vi "mqttCmdSend.vi"(0 "mqttBrokerCommand in":refnum<class "mqttCmd.lvclass">, 5 "byte1":u8, 7 "mqtt in":refnum<class "mqtt.lvclass">, 11 "error in (no error)":errorcluster) -> (4 "mqttBrokerCommand out":refnum<class "mqttCmd.lvclass">, 15 "error out":errorcluster)   [LabVIEW 2014, in "labview-mqtt.lvlib" / "mqttCmd.lvclass"]
uses:
  mqttCmd.lvclass
  mqtt.lvclass
  labview-mqtt.lvlib
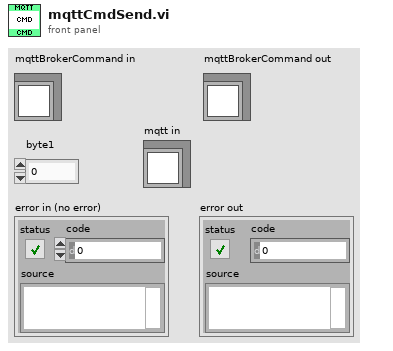
[diagram p1: front panel]
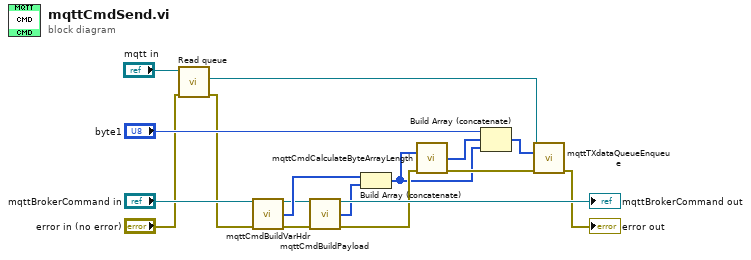
[diagram p0: block diagram]
diagram:
  n1 = call-dynamic "Read queue.vi"("error in (no error)"="error in (no error)", "mqtt in"="mqtt in") -> ("error out"=w1:errorcluster, "queue"=w3:refnum<queue>)  [unwired: 7 in, 1 out]
  n2 = call-dynamic "mqttCmdBuildVarHdr.vi"("_mqtt in"="mqttBrokerCommand in", "error in (no error)"=w1) -> ("_mqtt out"=w6:refnum<class "mqttCmd.lvclass">, "variableHeader"=w12:u8[], "error out"=w7:errorcluster)  [unwired: 11 in]
  n3 = call-dynamic "mqttCmdBuildPayload.vi"("_mqtt in"=w6, "error in (no error)"=w7) -> ("_mqtt out"=→"mqttBrokerCommand out":refnum<class "mqttCmd.lvclass">, "payload"=w13:u8[], "error out"=w11:errorcluster)  [unwired: 11 in]
  n4 = Build Array (concatenate)(w12, w13) -> (w10:u8[])
  n5 = call "mqttCmdCalculateByteArrayLength.vi"("byteArry in"=w10, "error in (no error)"=w11) -> ("length out"=w9:u8[], "error out"=w14:errorcluster)  [unwired: 12 in]
  n6 = Build Array (concatenate)("byte1", w9, w10) -> (w15:u8[])
  n7 = call "mqttTXdataQueueEnqueue.vi"("queue"=w3, "data in"=w15, "error in (no error)"=w14) -> ("error out"=→"error out":errorcluster)  [unwired: 12 in]
